vi "iRobot UART Bytes at Port.vi"(8 "error in":errorcluster, 11 "UART port in":T1) -> (0 "error out":errorcluster, 1 "bytes at port":u32, 3 "UART port out":T1)   [LabVIEW 2013]
doc: "Return the number of bytes in the UART receive buffer."
uses:
  iRobot UART Port Type.ctl
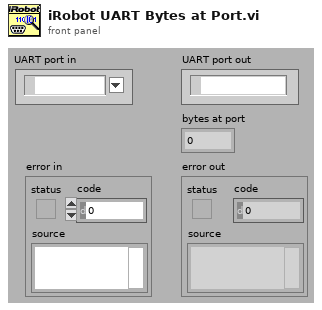
[diagram p1: front panel]
types:
  T1 = typedef "iRobot UART Port Type.ctl" = refnum<visa-resource-name>
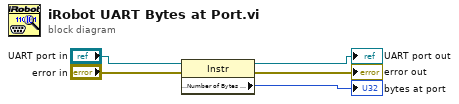
[diagram p0: block diagram]
diagram:
  n1 = property class="Instr"(reference="UART port in", error in="error in") -> (reference out=→"UART port out":T1, error out=→"error out":errorcluster, "Serial Settings:Number of Bytes at Serial Port"=→"bytes at port":u32)
